vi "Read Digital.vi"(7 "Slot Number (1)":u8=1 min=1 max=3 step=1, 8 "error in (no error)":errorcluster, 9 "Digital Port (F:1)":bool, 10 "Byte/Word (F:Byte)":bool, 11 "VISA Resource Name":refnum<visa-resource-name>) -> (0 "error out":errorcluster, 2 "Digital Value":bool[](array[boolean]), 3 "VISA Resource Name Out":refnum<visa-resource-name>)   [LabVIEW 2016, in "Agilent 34970.lvlib"]
doc: "This VI allows you to read a byte from one of the digital ports on the HP 34907A Multifunction module. Or, you can read a word from both ports simultaneously.\n\nThis is an advanced measurment VI. For more information on the different ways to take and configure a measurment, refer to the context help and block diagram of \"HP34970A Advanced Scan Example.vi\"."
uses:
  Agilent 34970.lvlib
panel:
  out "Message":string
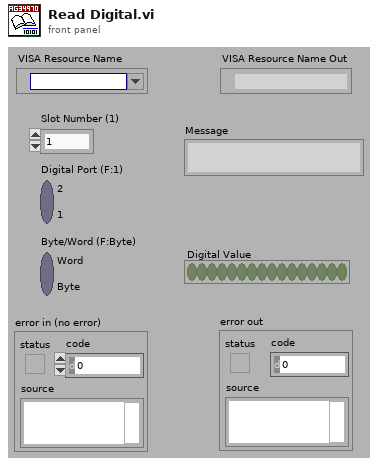
[diagram p1: front panel]
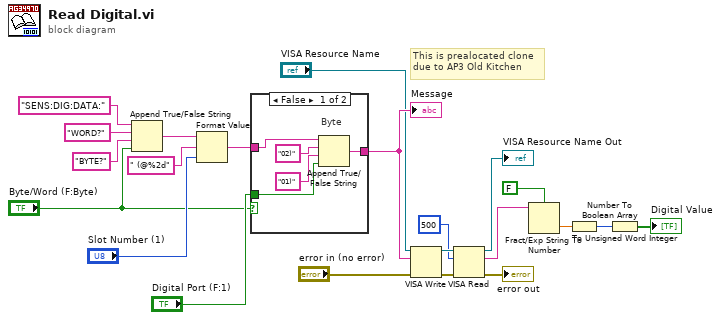
[diagram p0: block diagram]
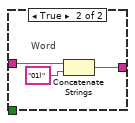
[diagram p2: hidden frame]
diagram:
  # "This is prealocated clone\ndue to AP3 Old Kitchen"
  n1 = Append True/False String(1:"Byte/Word (F:Byte)", 2:"BYTE?", 3:"WORD?", 4:"SENS:DIG:DATA:") -> (0:w2:string)
  n2 = Format Value(string ("")=w2, format string=" (@%2d", value (0)="Slot Number (1)") -> (output string=w11:string)
  n3 = case shown="False" "Byte/Word (F:Byte)" {
    tunnel: [w27 w29] -> w7
    tunnel: w11 -> [w26 w30]
    tunnel: "Digital Port (F:1)" -> [w23 _]
    frame False {
      # "Byte"
      n4 = Append True/False String(1:w23, 2:"01)", 3:"02)", 4:w26) -> (0:w27:string)
    }
    frame True {
      # "Word"
      n5 = Concatenate Strings(w30, "01)") -> (w29:string)
    }
  }
  "Message" <- w7
  n6 = VISA Write(VISA resource name="VISA Resource Name", write buffer=w7, error in (no error)="error in (no error)") -> (VISA resource name out=w19:refnum<visa-resource-name>, error out=w20:errorcluster)  [unwired: 1 out]
  n7 = VISA Read(VISA resource name=w19, byte count=u32 500 ("byte count (0)"), error in (no error)=w20) -> (VISA resource name out=→"VISA Resource Name Out":refnum<visa-resource-name>, read buffer=w14:string, error out=→"error out":errorcluster)  [unwired: 1 out]
  n8 = Fract/Exp String To Number(use system decimal point (T)=FALSE, string=w14) -> (number=w22:dbl)  [unwired: 2 in, 1 out]
  n9 = To Unsigned Word Integer(number=w22) -> (unsigned 16bit integer=w21:u16)
  n10 = Number To Boolean Array(number=w21) -> (Boolean array=→"Digital Value":bool[])
